vi "Read Scalar Shared Variables.vi"(8 "Error In":errorcluster, 9 "Array of Type code":i32[](array[numeric]), 10 "Array of SV Refnums":refnum<k21>[](array[refnum]), 11 "Waveform Array in":waveform(dbl)[](array[waveform])) -> (0 "Error Out":errorcluster, 3 "Waveform Array out":waveform(dbl)[](array[waveform]))   [LabVIEW 2014]
doc: "<B>Copyright</B>: (c) MHWirth 2015. All rights are reserved.\n\nThis subVI reads all shared variables (that are scalars), and consequently updates the input array of waveforms.\n\n<B>Shaved Variable Types</B>:\nType code 1 to 12 - \nIt does not support 1D or 2D arrays."
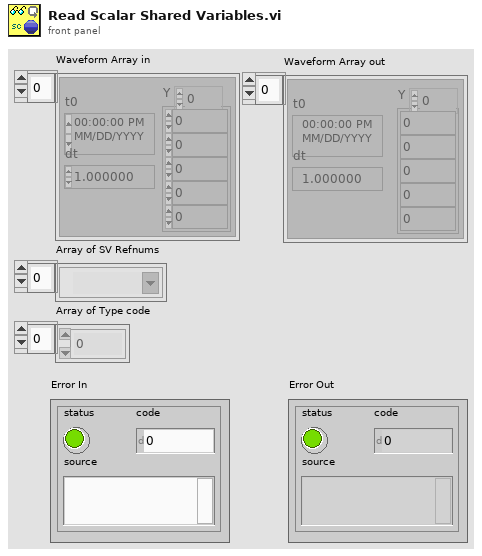
[diagram p1: front panel]
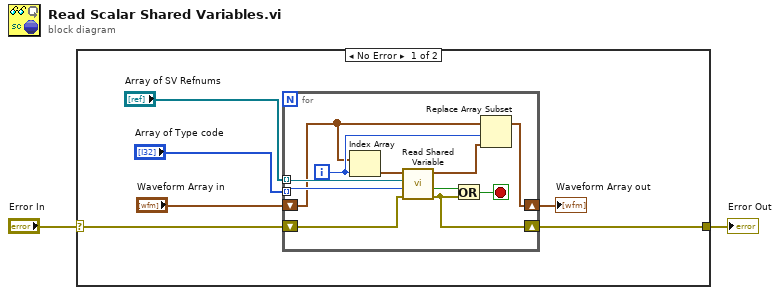
[diagram p0: block diagram]
diagram:
  n1 = case shown="No Error" "Error In" {
    selector: "Error In" -> [w4 w20]
    tunnel: [w3 w20] -> w2
    frame No Error {
      n2 = for {
        tunnel: "Array of SV Refnums" -> [w16] mode=indexing
        tunnel: "Array of Type code" -> [w17] mode=indexing
        shift-right: [w14] -> w3
        shift-left: w4 -> [w18]
        shift-right: [w9] -> w5
        shift-left: "Waveform Array in" -> [w10]
        i -> [w12]
        stop <- w19 stop-if-true
        n3 = Index Array(array=w10, index=w12) -> (element=w15:waveform(dbl))
        n4 = call "Read Shared Variable.vi"("Error In"=w18, "Type code"=w17, "Refnum"=w16, "Waveform in"=w15) -> ("Error Out"=w14:errorcluster, "status"=w13:bool, "Waveform out"=w11:waveform(dbl))  [unwired: 4 in, 1 out]
        n5 = Or(x=w13, y=w14) -> (x .or. y?=w19:bool)
        n6 = Replace Array Subset(array=w10, new element=w11, index=w12) -> (w9:waveform(dbl)[])
      }
      "Waveform Array out" <- w5
    }
    frame Error {
    }
  }
  "Error Out" <- w2
